vi "LWXPS_PositionerCompensationPostExcitationNotchModeFilterSet.vi"(0 "Positioner Name":string, 1 "Notch Mode Number":i32, 2 "Resonance frequency":dbl, 3 "Anti-resonance frequency":dbl, 4 "Resonance damping factor":dbl, 5 "Anti-resonance damping factor":dbl, 6 "XPS Reference IN":refnum<k24>, 7 "LabVIEW error IN":errorcluster) -> (14 "XPS Reference OUT":refnum<k24>, 15 "Returned error code":i32, 18 "XPS Error String":string, 19 "LabVIEW error OUT":errorcluster)   [LabVIEW 2014]
uses:
  D:/XPSQ8_LabView_Library/Development/Source/Dll/Newport.XPS.CommandInterface.dll
  Dll/Newport.XPS.CommandInterface.dll
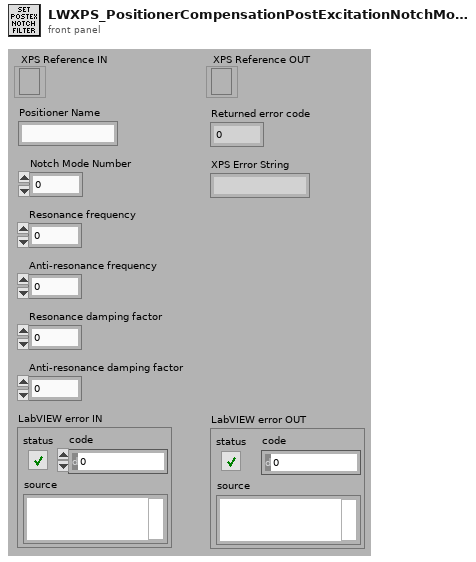
[diagram p1: front panel]
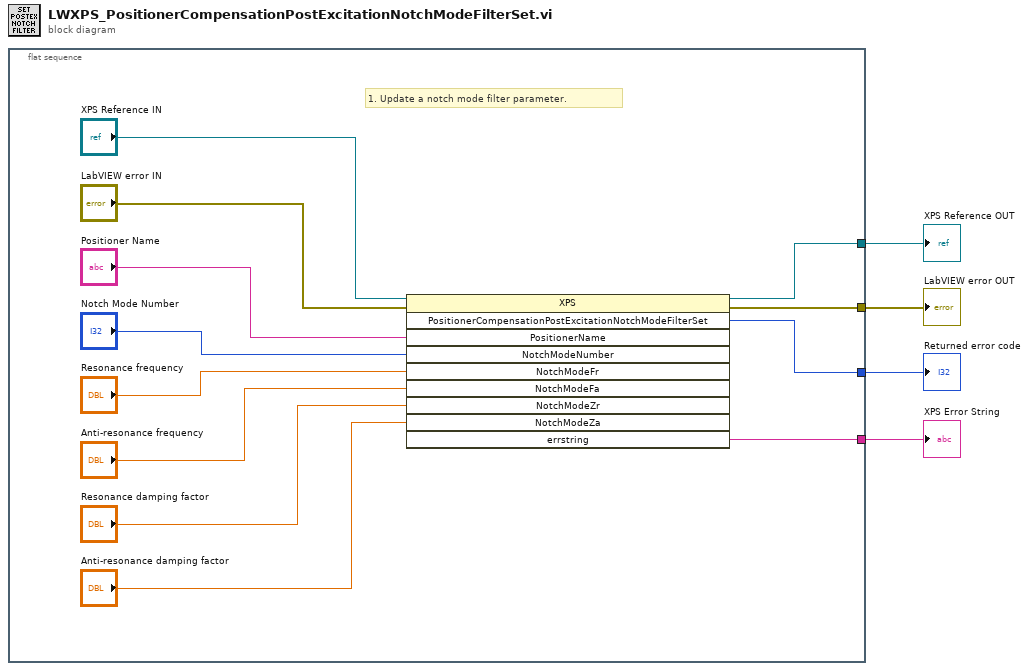
[diagram p0: block diagram]
diagram:
  n1 = flat-sequence {
    tunnel: [w12] -> w4
    tunnel: [w11] -> w3
    tunnel: [w13] -> w2
    tunnel: [w6] -> w1
    frame #0 {
      # "1. Update a notch mode filter parameter."
      n2 = invoke class="XPS" method="PositionerCompensationPostExcitationNotchModeFilterSet"(reference="XPS Reference IN", error in="LabVIEW error IN", "PositionerName"="Positioner Name", "NotchModeNumber"="Notch Mode Number", "NotchModeFr"="Resonance frequency", "NotchModeFa"="Anti-resonance frequency", "NotchModeZr"="Resonance damping factor", "NotchModeZa"="Anti-resonance damping factor") -> (reference out=w12:refnum<k24>, error out=w11:errorcluster, "PositionerCompensationPostExcitationNotchModeFilterSet"=w13:i32, "errstring"=w6:string)  [unwired: 2 in, 6 out]
    }
  }
  "XPS Error String" <- w1
  "XPS Reference OUT" <- w4
  "LabVIEW error OUT" <- w3
  "Returned error code" <- w2
